vi "Read Control.vi"(5 "High Address":u32 format="%08x", 7 "Base Address":u32 format="%08x", 11 "Address":u32 format="%08x") -> (0 "Error?":bool, 2 "Offset":u32 format="%08x", 3 "Data":i32 format="%08x")   [LabVIEW 2011]
uses:
  uBlaze VIVM Globals.vi
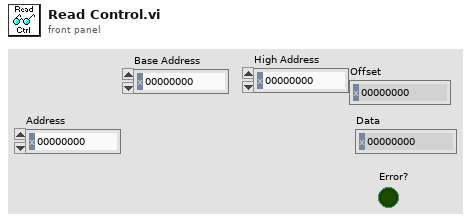
[diagram p1: front panel]
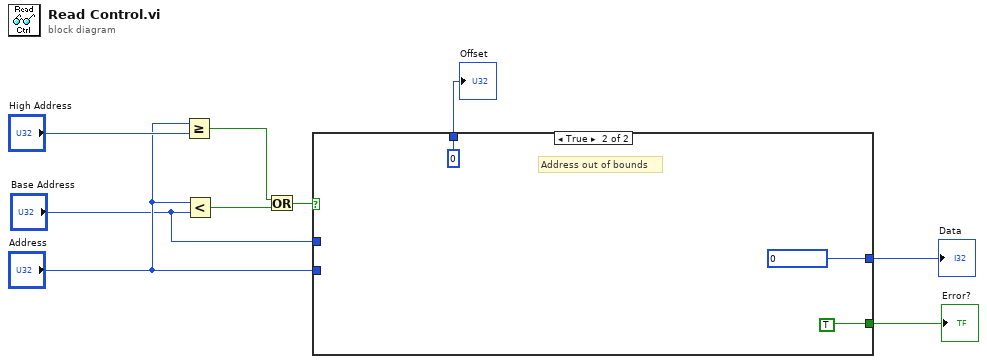
[diagram p0: block diagram]
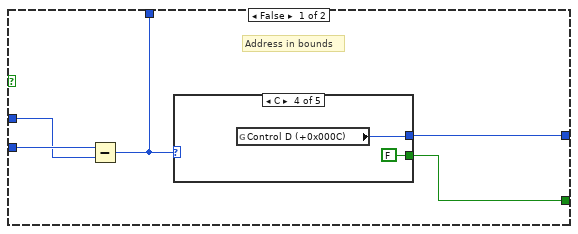
[diagram p2: hidden frame]
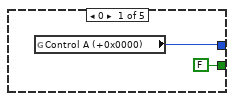
[diagram p3: hidden frame]
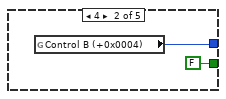
[diagram p4: hidden frame]
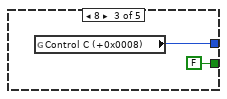
[diagram p5: hidden frame]
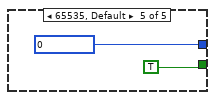
[diagram p6: hidden frame]
diagram:
  n1 = Greater Or Equal?(x="Address", y="High Address") -> (x >= y?=w3:bool)
  n2 = Less?(x="Address", y="Base Address") -> (x < y?=w2:bool)
  n3 = Or(x=w3, y=w2) -> (x .or. y?=w9:bool)
  n4 = case shown="True" w9 {
    tunnel: [w12 TRUE ("Error")] -> w7
    tunnel: "Address" -> [w14 _]
    tunnel: [w13 0 ("Data")] -> w5
    tunnel: [w11 u32 0] -> w4
    tunnel: "Base Address" -> [w10 _]
    frame False {
      # "Address in bounds"
      n5 = Subtract(x=w14, y=w10) -> (x-y=w11:u32)
      n6 = case shown="C" w11 {
        tunnel: [w16 w18 w20 w22 0 ("Data")] -> w13
        tunnel: [FALSE ("Error") FALSE ("Error") FALSE ("Error") FALSE ("Error") TRUE ("Error")] -> w12
        frame 0 {
          n7 = global read "uBlaze VIVM Globals.vi" "Control A (+0x0000)"() -> (w16:u32)
        }
        frame 4 {
          n8 = global read "uBlaze VIVM Globals.vi" "Control B (+0x0004)"() -> (w18:u32)
        }
        frame 8 {
          n9 = global read "uBlaze VIVM Globals.vi" "Control C (+0x0008)"() -> (w20:u32)
        }
        frame 12 {
          n10 = global read "uBlaze VIVM Globals.vi" "Control D (+0x000C)"() -> (w22:u32)
        }
        frame 65535, Default {
        }
      }
    }
    frame True {
      # "Address out of bounds"
    }
  }
  "Data" <- w5
  "Error?" <- w7
  "Offset" <- w4
